vi "ErrorMessage.vi"(1 "error in (no error)":errorcluster) -> (0 "Message String":string)   [LabVIEW 2025]
uses:
  <vilib>/Utility/error.llb/DialogType.ctl
  <userlib>/_OpenG.lib/string/string.llb/openg_string.lvlib
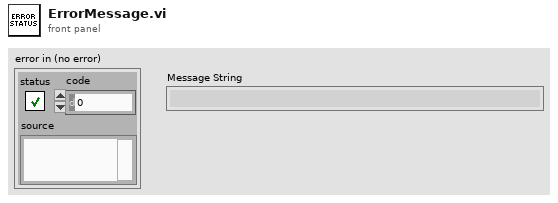
[diagram p1: front panel]
types:
  T1 = typedef "DialogType.ctl" = u16
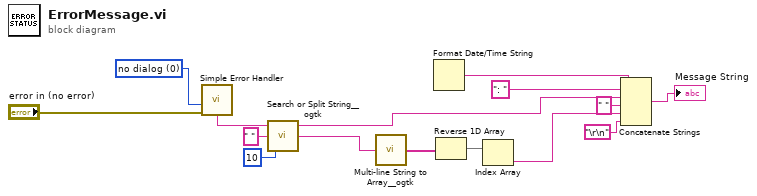
[diagram p0: block diagram]
diagram:
  w15 = T1 0 items=["no dialog", "OK message", "continue or stop message", "OK message + warnings", "continue/stop + warnings"] ("type of dialog (OK msg:1)")
  n1 = call <vilib>:"Simple Error Handler.vi"("type of dialog (OK msg:1)"=w15, "error in (no error)"="error in (no error)") -> ("message"=w14:string)  [unwired: 3 in, 4 out]
  n2 = call <userlib>:"Search or Split String__ogtk.vi"("offset (0)"=10, "search string/char (-)"=" ", "string"=w14) -> ("substring after match"=w11:string, "substring before match"=w6:string)  [unwired: 1 out]
  n3 = call <userlib>:"Multi-line String to Array__ogtk.vi"("string"=w11) -> ("lines"=w10:string[])
  n4 = Format Date/Time String() -> (date/time string=w8:string)  [unwired: 3 in]
  n5 = Reverse 1D Array(array=w10) -> (reversed array=w9:string[])
  n6 = Index Array(array=w9) -> (element=w5:string)  [unwired: 1 in]
  n7 = Concatenate Strings(w8, ": " ("string"), w6, " " ("string"), w5, "\r\n") -> (→"Message String":string)
